vi "XNET UDP Socket Close.vi"(8 "error in":errorcluster, 11 "socket":refnum<k20>) -> (0 "error out":errorcluster)   [LabVIEW 2018]
doc: "Closes a UDP socket and frees system resources."
uses:
  nixlvapi.dll
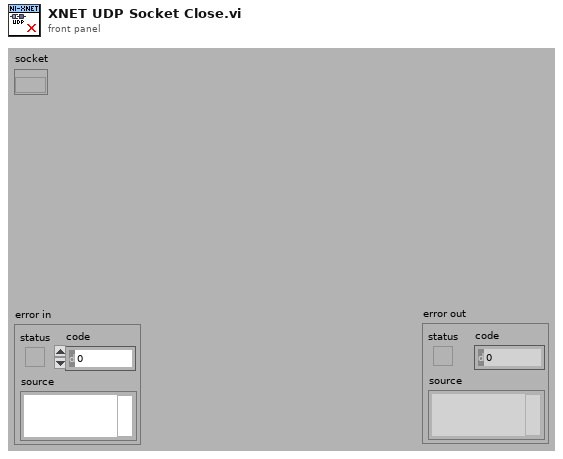
[diagram p1: front panel]
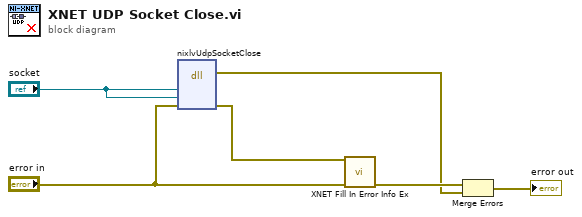
[diagram p0: block diagram]
diagram:
  n1 = dll-call lib="nixlvapi.*" fn="nixlvUdpSocketClose" label="Call Library"("socketRef"="socket", "socketRefObjPtr"="socket", "errorInOut"="error in") -> (error out=w4:errorcluster, "errorInOut"=w6:errorcluster)  [unwired: 3 in, 4 out]
  n2 = call "XNET Fill In Error Info Ex.vi"("error xnet"=w6, "error in"="error in") -> ("error out"=w5:errorcluster)  [unwired: 13 in]
  n3 = Merge Errors(w5, w4) -> (→"error out":errorcluster)
